vi "robust_scale.vi"(8 "error in":errorcluster caption="entrée d'erreur", 10 "X":string[][](array[string]), 11 "robust_scale":T2={"axis"=0, "with_centering"=TRUE, "with_scaling"=TRUE, "quantile_range"={"q_min"=25.0, "q_max"=75.0}, "copy"=TRUE}) -> (0 "error out":errorcluster caption="sortie d'erreur", 3 "Data":T1)   [LabVIEW 2020]
doc: "Standardize a dataset along any axis\n\nCenter to the median and component wise scale according to the interquartile range.\n\n\nParameters :\n\n- X : array-like\nThe data to center and scale.\n\n- axis : int (0 by default)\naxis used to compute the medians and IQR along. If 0, independently scale each feature, otherwise (if 1) scale each sample.\n\n- with_centering : boolean, True by default\nIf True, center the data before scaling.\n\n- with_scaling : boolean, True by default\nIf True, scale the data to unit variance (or equivalently, unit standard deviation).\n\n- quantile_range : tuple (q_min, q_max), 0.0 < q_min < q_max < 100.0\nDefault: (25.0, 75.0) = (1st quantile, 3rd quantile) = IQR Quantile range used to calculate scale_.\n\n- copy : boolean, optional, default is True\nset to False to perform inplace row normalization and avoid a copy (if the input is already a numpy array or a scipy.sparse CSR matrix and if axis is 1)."
uses:
  robust_scale.lvclass
panel:
  out "robust_scale.lvclass":refnum<class "robust_scale.lvclass">
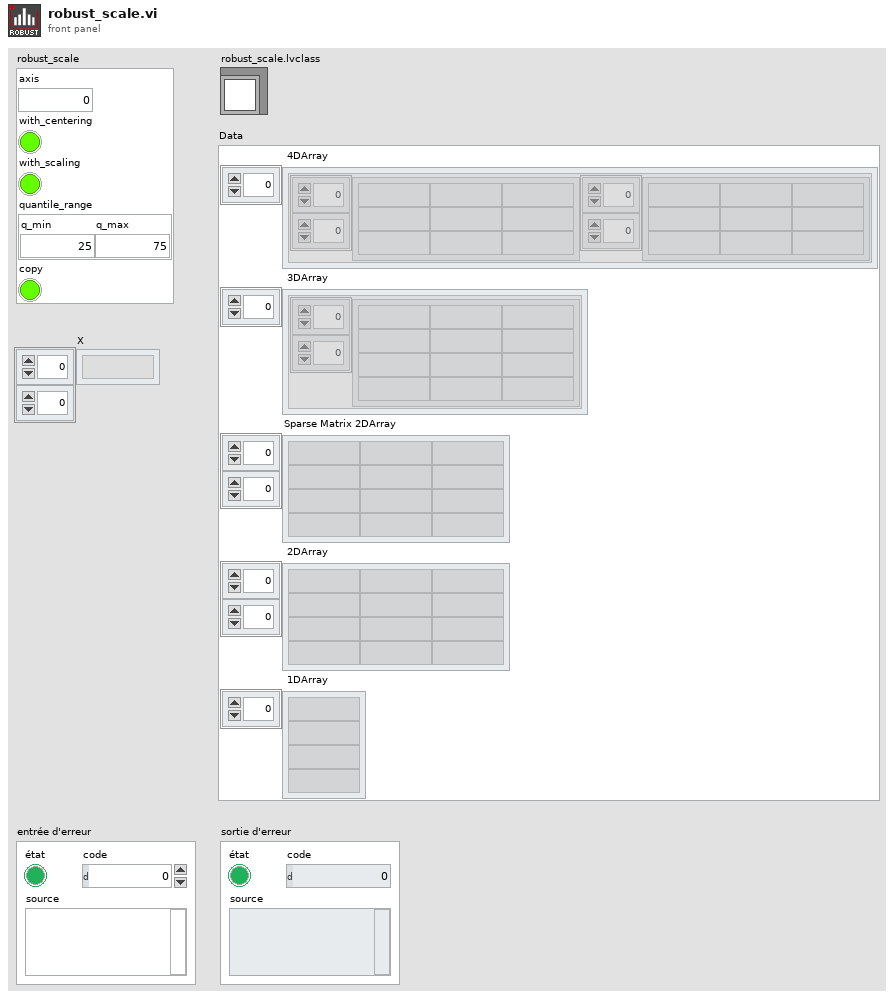
[diagram p1: front panel]
types:
  T1 = cluster{" 4DArray":cluster{"1":string[][], "2":string[][]}[], " 3DArray":cluster{"Tableau":string[][]}[], "Sparse Matrix 2DArray":string[][], " 2DArray":string[][], " 1DArray":string[]}
  T2 = cluster{"axis":i32, "with_centering":bool, "with_scaling":bool, "quantile_range":cluster{"q_min":dbl, "q_max":dbl}, "copy":bool}
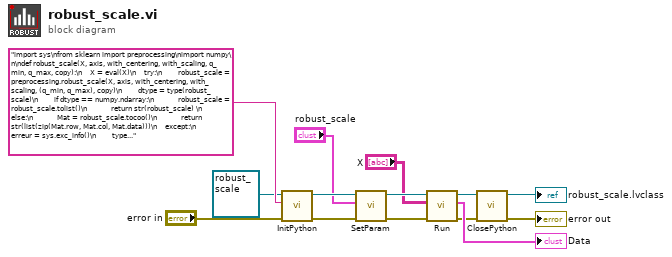
[diagram p0: block diagram]
diagram:
  n1 = call-dynamic "InitPython.vi"("error in (no error)"="error in", "Python Instruction"="import sys\nfrom sklearn import preprocessing\nimport numpy\n\ndef robust_scale(X, axis, with_centering, with_scaling, q_min, q_max, copy):\n    X = eval(X)\n    try:\n        robust_scale = preprocessing.robust_scale(X, axis, with_centering, with_scaling, (q_min, q_max), copy)\n        dtype = type(robust_scale)\n        if dtype == numpy.ndarray:\n            robust_scale = robust_scale.tolist()\n            return str(robust_scale) \n        else:\n            Mat = robust_scale.tocoo()\n            return str(list(zip(Mat.row, Mat.col, Mat.data)))\n    except:\n        erreur = sys.exc_info()\n        typerr = u\"%s\" % (erreur[0])\n        typerr = typerr[typerr.find(\"'\")+1:typerr.rfind(\"'\")]\n        msgerr = u\"%s\" % (erreur[1])\n        message = str('/!\\\\ {0} : {1}'. format(typerr,msgerr))\n        return message", "Scikit-learn en entrée"=refnum<class "robust_scale.lvclass"> refnum ("robust_scale.lvclass")) -> ("error out"=w9:errorcluster, "Scikit-learn en sortie"=w10:refnum<class "robust_scale.lvclass">)  [unwired: 7 in]
  n2 = call-dynamic "SetParam.vi"("error in (no error)"=w9, "robust_scale"="robust_scale", "robust_scale.lvclass"=w10) -> ("error out"=w6:errorcluster, "robust_scale.lvclass"=w7:refnum<class "robust_scale.lvclass">)  [unwired: 7 in]
  n3 = call-dynamic "Run.vi"("error in (no error)"=w6, "X"="X", "robust_scale.lvclass"=w7) -> ("error out"=w3:errorcluster, "Data"=→"Data":T1, "robust_scale.lvclass"=w5:refnum<class "robust_scale.lvclass">)  [unwired: 6 in]
  n4 = call-dynamic "ClosePython.vi"("error in (no error)"=w3, "Scikit-learn en entrée"=w5) -> ("error out"=→"error out":errorcluster, "Scikit-learn en sortie"=→"robust_scale.lvclass":refnum<class "robust_scale.lvclass">)  [unwired: 8 in]
